vi "LWXPS_GPIOAnalogGet.vi"(8 "LabVIEW error IN":errorcluster, 10 "GPIO Name IN":string[](array[string]), 11 "XPS Reference IN":refnum<k24>) -> (0 "XPS Error String":string, 1 "Analog Value":dbl[](array[numeric]), 2 "GPIO Name OUT":string[](array[string]), 3 "Returned error code":i32, 4 "LabVIEW error OUT":errorcluster, 5 "XPS Reference OUT":refnum<k24>)   [LabVIEW 2014]
uses:
  D:/XPSQ8_LabView_Library/Development/Source/Dll/Newport.XPS.CommandInterface.dll
  Dll/Newport.XPS.CommandInterface.dll
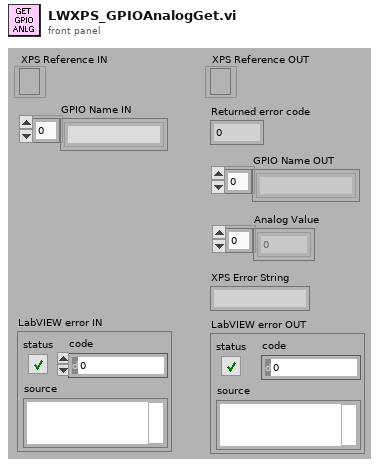
[diagram p1: front panel]
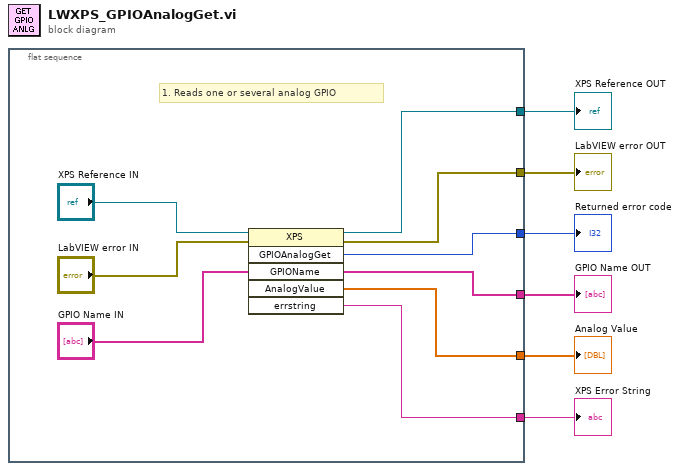
[diagram p0: block diagram]
diagram:
  n1 = flat-sequence {
    tunnel: [w11] -> w6
    tunnel: [w14] -> w5
    tunnel: [w12] -> w4
    tunnel: [w9] -> w1
    tunnel: [w10] -> w2
    tunnel: [w8] -> w3
    frame #0 {
      # "1. Reads one or several analog GPIO"
      n2 = invoke class="XPS" method="GPIOAnalogGet"(reference="XPS Reference IN", error in="LabVIEW error IN", "GPIOName"="GPIO Name IN") -> (reference out=w11:refnum<k24>, error out=w14:errorcluster, "GPIOAnalogGet"=w12:i32, "GPIOName"=w10:string[], "AnalogValue"=w9:dbl[], "errstring"=w8:string)  [unwired: 3 in]
    }
  }
  "XPS Reference OUT" <- w6
  "LabVIEW error OUT" <- w5
  "Returned error code" <- w4
  "XPS Error String" <- w3
  "GPIO Name OUT" <- w2
  "Analog Value" <- w1
